vi "PCO_SetDelayExposureTimeTable.vi"(0 "ph":u64, 1 "wTimeBaseExposure":u16(ring) items=["ns", "us", "ms"], 5 "dwDelay":u32[](array[numeric])=array[4097 elements], 7 "dwExposure":u32[](array[numeric])=array[4097 elements], 9 "wTimeBaseDelay":u16(ring) items=["ns", "us", "ms"], 11 "error in (no error)":errorcluster {"code" format="%x"}) -> (4 "ph out":u64, 6 "ErrorMessage":i32 format="%x", 15 "error out":errorcluster {"code" format="%x"})   [LabVIEW 2019, in "SDK.lvlib" / "TimingControl.lvlib"]
doc: "<b>Description:</b>\nThis function does set the delay and exposure time pairs in the time tables and the associated time base values. Maximum size of each table array is 16 DWORD entries. Delay / exposure time table operation is supported, if wTimeTableDESC in the camera description is set. After the camera is started it will take a series of consecutive images with delay and exposure times, as defined in the table. The first found exposure time entry with value zero does break the sequence and operation starts again from the beginning of the table. This results in a sequence of 1 to 16 images with different delay and exposure time settings. External or automatic image triggering is fully functional for every image in the sequence. If the user wants maximum speed (at CCDs overlapping exposure and read out is taken), [auto trigger] should be selected and the sequence should be controlled with the <acq enbl> input.\nThe commands PCO_SetDelayExposureTime and PCO_SetDelayExposureTimeTable can only be used alternatively. Using PCO_SetDelayExposureTime has the same effect as using the PCO_SetDelayExposureTimeTable command and setting all but the first delay / exposure entry to zero.\n\nRestrictions for the parameter values are defined through the following values in the camera description PCO_Description structure: dwMinDelayDESC, dwMaxDelayDESC, dwMinDelayStepDESC, dwMinExposDESC, dwMaxExposDESC, dwMinExposStepDESC\n\n<b>Supported camera type:</b>\nAll cameras\n\n<b>Descriptor dependency:</b>\nwTimeTableDESC"
uses:
  TimingControl.lvlib
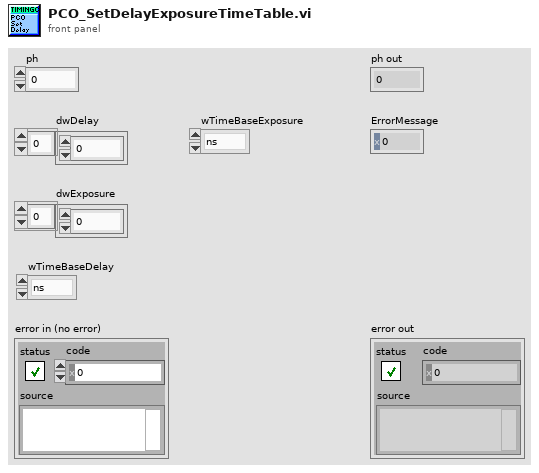
[diagram p1: front panel]
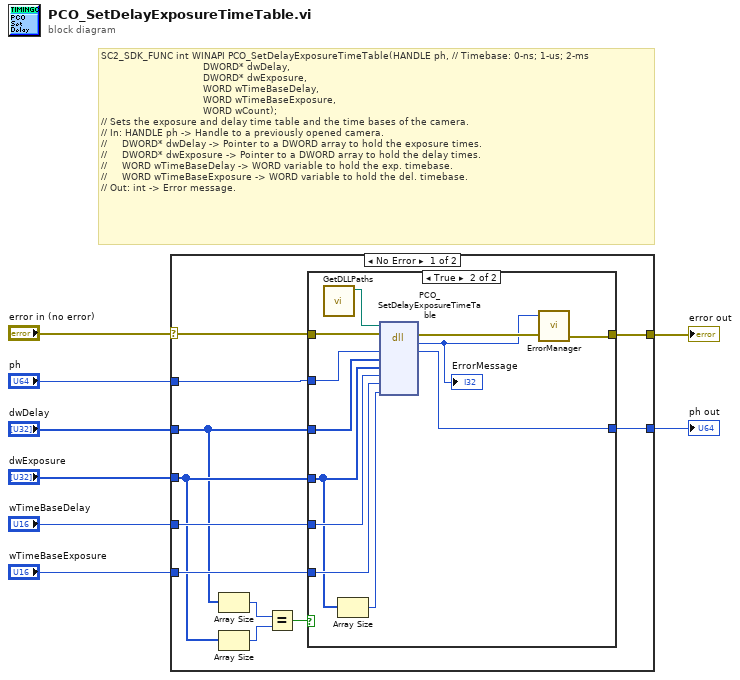
[diagram p0: block diagram]
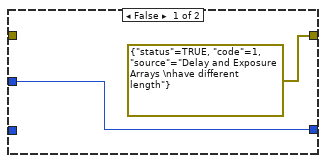
[diagram p2: hidden frame]
diagram:
  # "SC2_SDK_FUNC int WINAPI PCO_SetDelayExposureTimeTable(HANDLE ph, // Timebase: 0-ns; 1-us; 2-ms \n                                  DWORD* dwDelay,\n                                  DWORD* dwExposure,\n                                  WORD wTimeBaseDelay,\n                                  WORD wTimeBaseExposure,\n                                  WORD wCount);\n// Sets the exposure and delay time table and the time bases of the camera.\n// In: HANDLE ph -> Handle to a previously opened camera.\n//     DWORD* dwDelay -> Pointer to a DWORD array to hold the exposure times.\n//     DWORD* dwExposure -> Pointer to a DWORD array to hold the delay times.\n//     WORD wTimeBaseDelay -> WORD variable to hold the exp. timebase.\n//     WORD wTimeBaseExposure -> WORD variable to hold the del. timebase.\n// Out: int -> Error message."
  n1 = case shown="No Error" "error in (no error)" {
    selector: "error in (no error)" -> [w13 w35]
    tunnel: "ph" -> [w10 w34]
    tunnel: [w19 w34] -> w7
    tunnel: "wTimeBaseDelay" -> [w18 _]
    tunnel: "wTimeBaseExposure" -> [w17 _]
    tunnel: [w16 w35] -> w4
    tunnel: "dwExposure" -> [w15 _]
    tunnel: "dwDelay" -> [w14 _]
    frame No Error {
      n2 = Array Size(array=w14) -> (size(s)=w11:i32)
      n3 = Array Size(array=w15) -> (size(s)=w12:i32)
      n4 = Equal?(x=w11, y=w12) -> (x = y?=w9:bool)
      n5 = case shown="True" w9 {
        tunnel: [w21 w33] -> w19
        tunnel: w18 -> [_ w32]
        tunnel: w17 -> [_ w31]
        tunnel: [errorcluster {"status"=TRUE, "code"=1, "source"="Delay and Exposure Arrays \nhave different length"} ("error out") w24] -> w16
        tunnel: w15 -> [_ w27]
        tunnel: w14 -> [_ w30]
        tunnel: w13 -> [_ w29]
        tunnel: w10 -> [w21 w28]
        frame False {
        }
        frame True {
          n6 = call "GetDLLPaths.vi"() -> ("SC2_Cam_Path"=w22:path)  [unwired: 8 in, 3 out]
          n7 = Array Size(array=w27) -> (size(s)=w26:i32)
          n8 = dll-call lib="?" fn="PCO_SetDelayExposureTimeTable"(path in=w22, error in=w29, "ph"=w28, "dwDelay"=w30, "dwExposure"=w27, "wTimeBaseDelay"=w32, "wTimeBaseExposure"=w31, "wCount"=w26) -> (error out=w25:errorcluster, "return type"=w23:i32, "ph"=w33:u64)  [unwired: 6 in, 1 out]
          "ErrorMessage" <- w23
          n9 = call "ErrorManager.vi"("error in (no error)"=w25, "error code"=w23) -> ("error out"=w24:errorcluster)  [unwired: 2 in, 1 out]
        }
      }
    }
    frame Error {
    }
  }
  "ph out" <- w7
  "error out" <- w4
